vi "0-Helper-Overlay Circle.vi"(6 "Radius (px)":dbl, 9 "Pixel Coordinates":cluster{"X":i32, "Y":i32}, 10 "Color":u32(colorbox)=16754450, 11 "Image in":T1) -> (3 "Image out":T1)   [LabVIEW 2011]
doc: "Overlays an unfilled circle on the input image, with the given radius and location, in pixels, and the given color."
uses:
  <vilib>/vision/Image Controls.llb/IMAQ Image.ctl
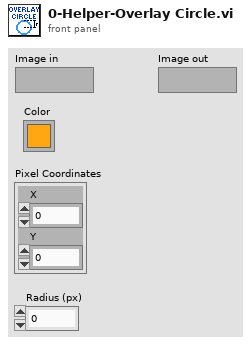
[diagram p1: front panel]
types:
  T1 = typedef "IMAQ Image.ctl" = refnum<image>
  T2 = cluster{"Left":i32, "Top":i32, "Right":i32, "Bottom":i32}
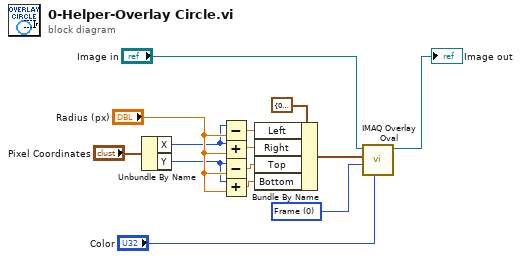
[diagram p0: block diagram]
diagram:
  w2 = u32 0 items=["Frame", "Fill"] ("Drawing Mode (Frame)")
  n1 = Unbundle By Name("Pixel Coordinates") -> ("X"=w9:i32, "Y"=w10:i32)
  n2 = Subtract(x=w9, y="Radius (px)") -> (x-y=w5:dbl)
  n3 = Add(x=w9, y="Radius (px)") -> (x+y=w4:dbl)
  n4 = Subtract(x=w10, y="Radius (px)") -> (x-y=w7:dbl)
  n5 = Add(x=w10, y="Radius (px)") -> (x+y=w6:dbl)
  n6 = Bundle By Name(cluster=T2 {"Left"=0, "Top"=0, "Right"=0, "Bottom"=0} ("Bounding Rectangle"), "Left"=w5, "Right"=w4, "Top"=w7, "Bottom"=w6) -> (w12:T2)
  n7 = call "IMAQ Overlay Oval"("Color"="Color", "Drawing Mode (Frame)"=w2, "Bounding Rectangle"=w12, "Image"="Image in") -> ("Image Out"=→"Image out":T1)  [unwired: 6 in, 1 out]
